vi "MAVLink Battery.vi"(7 "FGV Method":T2, 11 "Battery Info":T1 {"Batt Voltage (V)" format="%.2f"; "Batt Current (Ah)" format="%.2f"}) -> (3 "Battery Info out":T1 {"Batt Voltage (V)" format="%.2f"; "Batt Current (Ah)" format="%.2f"})   [LabVIEW 2014]
uses:
  Controls/FGV Methods.ctl
  MAVLink/Controls/MAVLink Battery.ctl
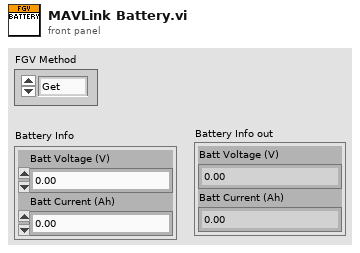
[diagram p1: front panel]
types:
  T1 = typedef "MAVLink Battery.ctl" = cluster{"Batt Voltage (V)":dbl, "Batt Current (Ah)":dbl}
  T2 = typedef "FGV Methods.ctl" = enum16{"Get", "Set"}
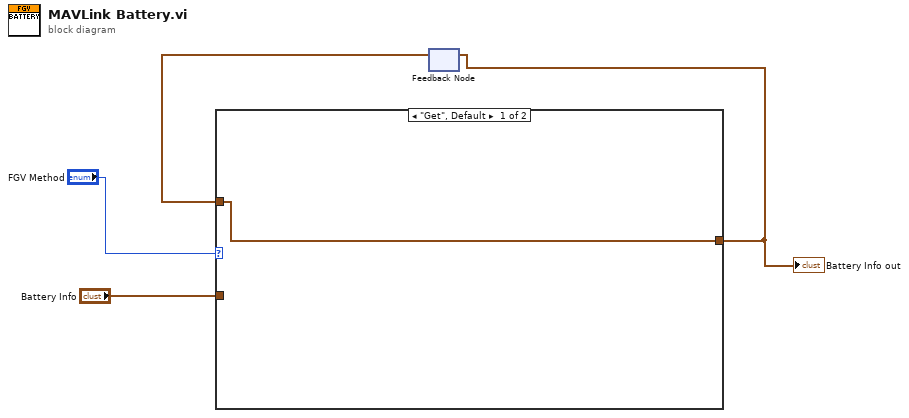
[diagram p0: block diagram]
diagram:
  n1 = feedback #1() -> (w2:T1)  [unwired: 1 in]
  n2 = case shown="\"Get\", Default" "FGV Method" {
    tunnel: "Battery Info" -> [_ w6]
    tunnel: [w5 w6] -> w3
    tunnel: w2 -> [w5 _]
    frame "Get", Default {
    }
    frame "Set" {
    }
  }
  "Battery Info out" <- w3
  n3 = feedback-in #1(w3) -> ()
